vi "Sort Landmarks.vi"(8 "error in (no error)":errorcluster, 10 "SLAM In":T1) -> (0 "error out":errorcluster, 2 "SLAM Out":T1)   [LabVIEW 2009]
uses:
  Controls/SLAM.ctl
  <vilib>/Analysis/Matrix/Datatypes/RealMatrix.ctl
  <vilib>/Analysis/Matrix/NI_Matrix.lvlib
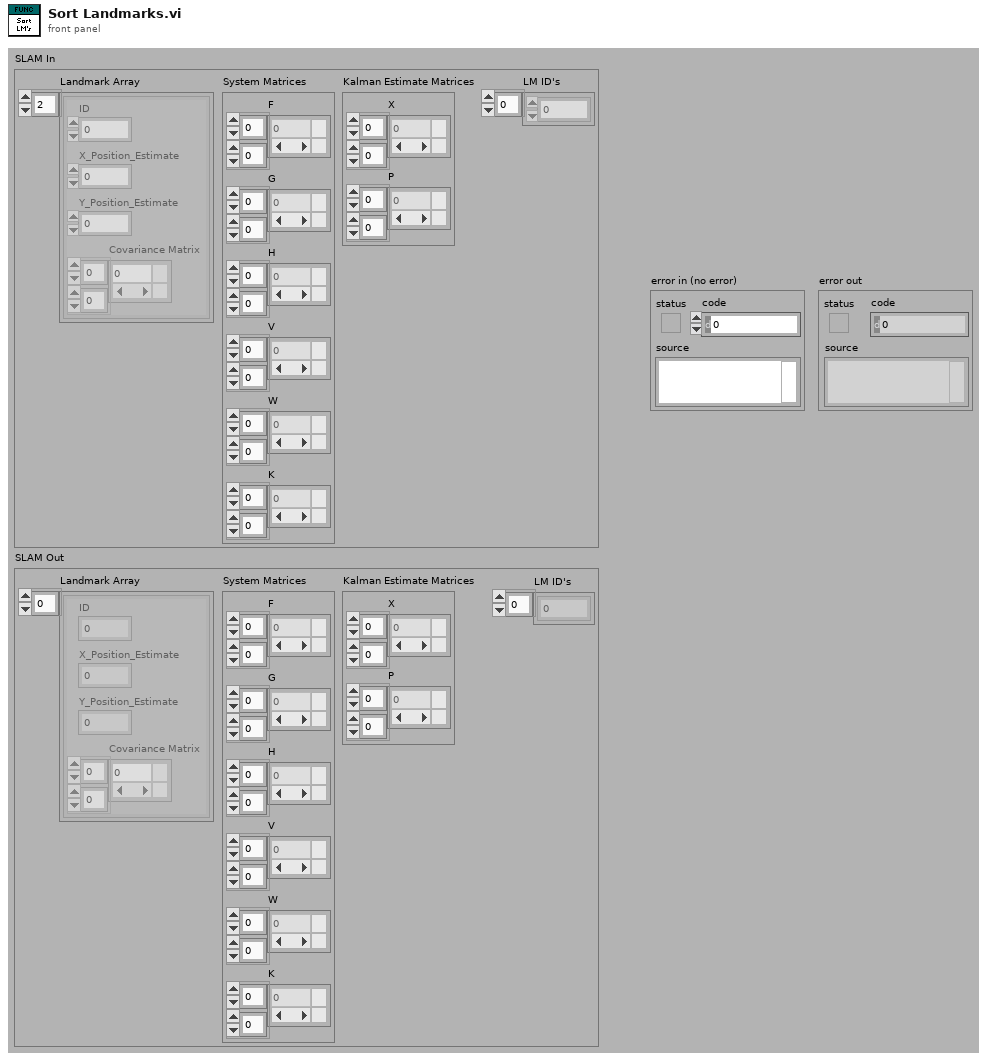
[diagram p1: front panel]
types:
  T1 = typedef "SLAM.ctl" = cluster{"Landmark Array":cluster{"ID":dbl, "X_Position_Estimate":dbl, "Y_Position_Estimate":dbl, "Covariance Matrix":T2}[], "System Matrices":cluster{"F":T2, "G":T2, "H":T2, "V":T2, "W":T2, "K":T2}, "Kalman Estimate Matrices":cluster{"X":T2, "P":T2}, "LM ID's":dbl[]}
  T2 = typedef "NI_Matrix.lvlib/RealMatrix.ctl" = dbl[][]
  T3 = cluster{"ID":dbl, "X_Position_Estimate":dbl, "Y_Position_Estimate":dbl, "Covariance Matrix":T2}[]
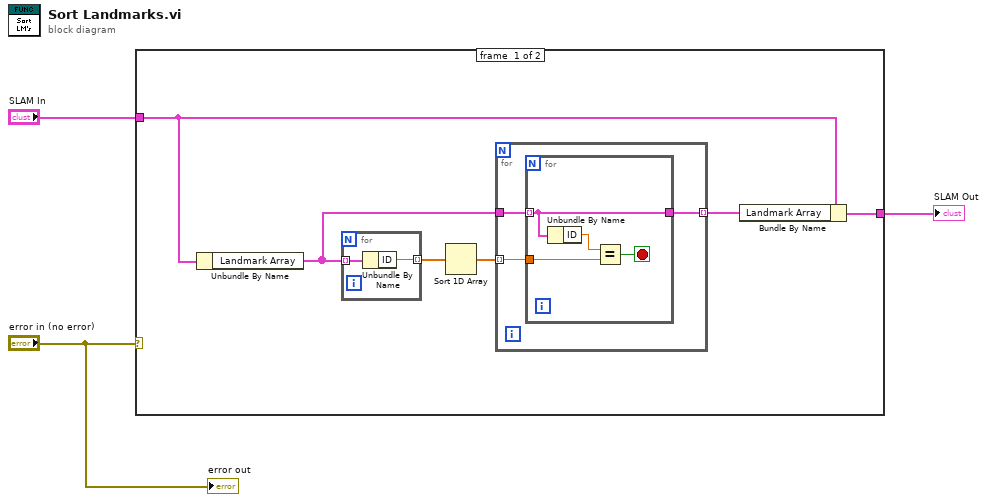
[diagram p0: block diagram]
diagram:
  n1 = case shown="No Error" "error in (no error)" {
    tunnel: "SLAM In" -> [w6 w19]
    tunnel: [w5 w19] -> w2
    frame #0 {
      n2 = Unbundle By Name(w6) -> ("Landmark Array"=w7:T3)
      n3 = for {
        tunnel: w7 -> [w18] mode=indexing
        tunnel: [w17] -> w9 mode=indexing
        n4 = Unbundle By Name(w18) -> ("ID"=w17:dbl)
      }
      n5 = Sort 1D Array(array=w9) -> (sorted array=w8:dbl[])
      n6 = for {
        tunnel: w8 -> [w12] mode=indexing
        tunnel: w7 -> [w11]
        tunnel: [w10] -> w4 mode=indexing
        n7 = for {
          tunnel: w12 -> [w15]
          tunnel: w11 -> [w13] mode=indexing
          tunnel: [w13] -> w10
          stop <- w14 stop-if-true
          n8 = Unbundle By Name(w13) -> ("ID"=w16:dbl)
          n9 = Equal?(x=w16, y=w15) -> (x = y?=w14:bool)
        }
      }
      n10 = Bundle By Name(cluster=w6, "Landmark Array"=w4) -> (w5:T1)
    }
    frame #1 {
    }
  }
  "SLAM Out" <- w2
  "error out" <- "error in (no error)"
